vi "gg.vi"   [LabVIEW 2017]
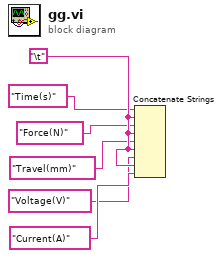
[diagram p0: block diagram]
diagram:
  w5 = "\t"
  n1 = Concatenate Strings("Time(s)", w5, "Force(N)", w5, "Travel(mm)", w5, "Voltage(V)", w5, "Current(A)") -> ()  [unwired: 1 out]
